vi "register put.vi"(8 "error in (no error)":errorcluster, 10 "register address":i32) -> (0 "error out":errorcluster)   [LabVIEW 2019]
uses:
  servo state.ctl
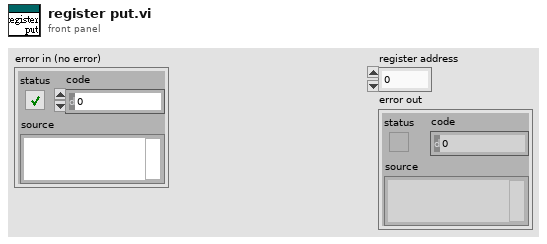
[diagram p1: front panel]
types:
  T1 = typedef "servo state.ctl" = enum16{"catch", "cam-1", "put", "side", "center", "side-2", "put-2"}
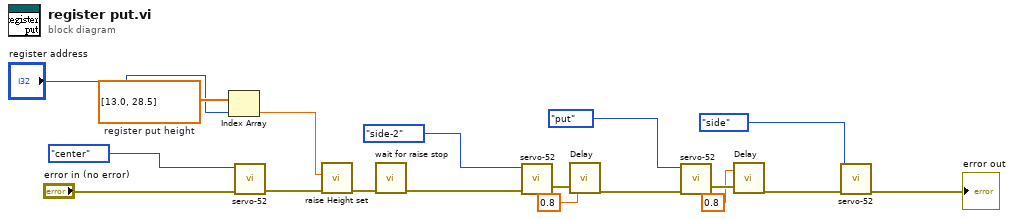
[diagram p0: block diagram]
diagram:
  w16 = dbl[] [13.0, 28.5]  # register put height
  n1 = Index Array(array=w16, index="register address") -> (element=w13:dbl)
  n2 = call "servo-52.vi"("error in (no error)"="error in (no error)", "Enum"=servo_state."center") -> ("error out"=w14:errorcluster)  [unwired: 9 in]
  n3 = call "raise Height set.vi"("error in (no error)"=w14, "Height_cm"=w13) -> ("error out"=w12:errorcluster)  [unwired: 9 in]
  n4 = call "wait for raise stop.vi"("Error In"=w12) -> ("Error Out"=w11:errorcluster)  [unwired: 10 in]
  n5 = call "servo-52.vi"("error in (no error)"=w11, "Enum"=servo_state."side-2") -> ("error out"=w9:errorcluster)  [unwired: 9 in]
  n6 = call "Delay.vi"("error in (no error)"=w9, "Delay Time (s)"=0.8) -> ("error out"=w8:errorcluster)  [unwired: 1 in]
  n7 = call "servo-52.vi"("error in (no error)"=w8, "Enum"=servo_state."put") -> ("error out"=w6:errorcluster)  [unwired: 9 in]
  n8 = call "Delay.vi"("error in (no error)"=w6, "Delay Time (s)"=0.8) -> ("error out"=w5:errorcluster)  [unwired: 1 in]
  n9 = call "servo-52.vi"("error in (no error)"=w5, "Enum"=servo_state."side") -> ("error out"=→"error out":errorcluster)  [unwired: 9 in]
